vi "I(V) at various fields_MFLI_PK_v4.0_measure X.vi"() -> ()   [LabVIEW 2016]
uses:
  Labview Drivers/MFLI/LabOneLabVIEW-22.02.26577/LabOneLabVIEW-22.02.26577/Zurich Instruments LabOne/Public/Data/ziTypeDemodSampleSingle.ctl
  Labview Drivers/MFLI/LabOneLabVIEW-22.02.26577/LabOneLabVIEW-22.02.26577/Zurich Instruments LabOne/Public/Configure/ziSetValueDouble.vi
  Labview Drivers/MFLI/LabOneLabVIEW-22.02.26577/LabOneLabVIEW-22.02.26577/Zurich Instruments LabOne/Public/Configure/ziGetValueDemodSampleEx.vi
  Labview Drivers/MFLI/LabOneLabVIEW-22.02.26577/LabOneLabVIEW-22.02.26577/Zurich Instruments LabOne/Zurich Instruments LabOne.lvlib
panel:
  out "Time (s)":dbl format="%#_13g"
  in  "Field ramp rate (T/min)":string="0.05"
  in  "Magnetic field stabilization time (s)":dbl=200.0 format="%#_13g"
  in  "Step 2":dbl[](array[numeric])=[0.25] min=-3000.0 max=3000.0 format="%.1e"
  in  "To 2":dbl[](array[numeric])=[6.0] min=-3000.0 max=3000.0 format="%.1e"
  in  "From 2":dbl[](array[numeric])=[8.5] min=-3000.0 max=3000.0 format="%.1e"
  out "Magnetic Field (T)":dbl format="%#_13g"
  in  "Magnet IP Address":string="169.254.46.132"
  out "Demod Sample Out 2":T1={"Timestamps (ticks)"=34359738372, "X (Vrms)"=8.366245757779461e-285, "Y (Vrms)"=1.0096057436928657e-284, "Osc Phase (deg)"=1.69759663376e-313, "Freq (Hz)"=2.607691286315397e-191, "DIO"=4, "AuxIn0 (V)"=0.0, "AuxIn1 (V)"=1.6954746369817e-311, "Trigger"=16}
  out "Demod Sample Out":T1={"Timestamps (ticks)"=34359738372, "X (Vrms)"=8.366245757779461e-285, "Y (Vrms)"=1.0096057436928657e-284, "Osc Phase (deg)"=1.69759663376e-313, "Freq (Hz)"=2.607691286315397e-191, "DIO"=4, "AuxIn0 (V)"=0.0, "AuxIn1 (V)"=1.6954746369817e-311, "Trigger"=16}
  in  "MFLI Current source/Voltage reader":string="DEV4382"
  out "Imeas (A)":dbl=2.528615115e-315
  out "Vmeas (V)":dbl=nan
  in  "Folder":path=path "D:/Pranava/Data/NbO/27-05-2020"
  in  "MFLI stabilization time (s) [> TC]":u32=1
  out "I vs V":cluster{dbl, "Field Reading":dbl}[](graph)=[{nan, "Field Reading"=3.54694038e-315}, {nan, "Field Reading"=2.528615115e-315}]
  out "data":dbl[](array[numeric])=[nan, 2.528615115e-315, 0.0001]
  in  "Step":dbl[](array[numeric])=[0.001, 0.001, 0.001] min=-3000.0 max=3000.0 format="%.1e"
  in  "To":dbl[](array[numeric])=[0.5, -0.5, 0.0] min=-3000.0 max=3000.0 format="%.1e"
  in  "From":dbl[](array[numeric])=[0.0, 0.5, -0.5] min=-3000.0 max=3000.0 format="%.1e"
  in  "file name":string="001_IV_(Nb)STO_7mK_MFLI_MF-MD"
  out "File path":path=path "D:/Pranava/Data/001_IV_(Nb)STO_7mK_MFLI_MF-MD.dat"
  # ".dat"
  # "[Must be less than 0.05]"
  # "Set MFLI Voltage output (V)"
  # "Configure Magnetic field sweep (T)"
types:
  T1 = typedef "Zurich Instruments LabOne.lvlib/ziTypeDemodSampleSingle.ctl" = cluster{"Timestamps (ticks)":u64, "X (Vrms)":dbl, "Y (Vrms)":dbl, "Osc Phase (deg)":dbl, "Freq (Hz)":dbl, "DIO":u32, "AuxIn0 (V)":dbl, "AuxIn1 (V)":dbl, "Trigger":u32}
  T2 = enum16{"open", "replace", "create", "open or create", "replace or create", "replace or create with confirmation"}
  T3 = typedef "Zurich Instruments LabOne.lvlib/ziTypeHandle.ctl" = cluster{"handleValid":bool, "Conn":u64, "Path Prefix":string, "Handle":u64, "Connected":bool, "Clockbase(s)":dbl}
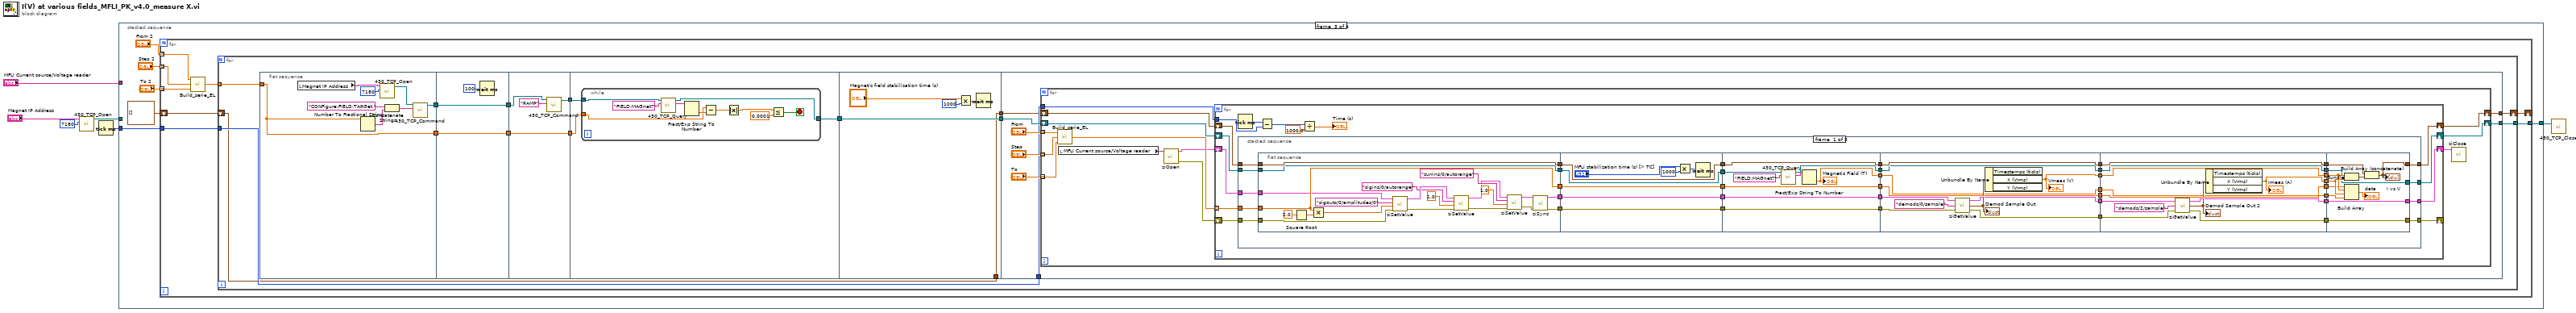
[diagram p0: block diagram]
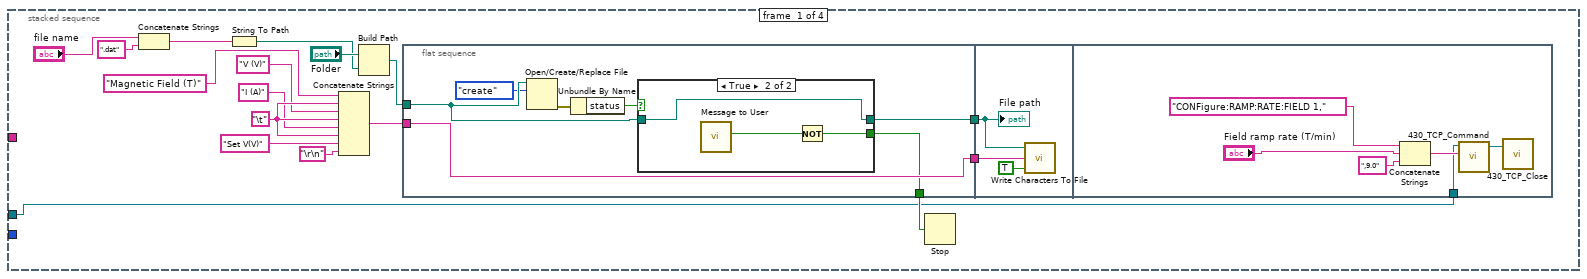
[diagram p2: hidden frame]
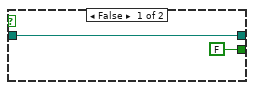
[diagram p3: hidden frame]
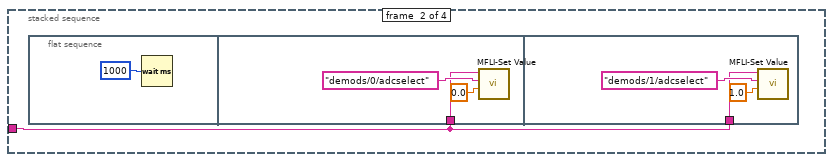
[diagram p4: hidden frame]
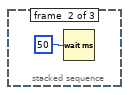
[diagram p5: hidden frame]
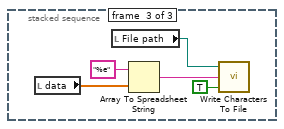
[diagram p6: hidden frame]
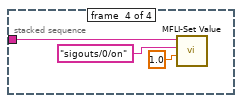
[diagram p7: hidden frame]
diagram:
  n1 = call "430_TCP_Open.vi"("IP Address"="Magnet IP Address", "TCP Port"=7180) -> ("connection ID"=w2:refnum<k5>)  [unwired: 4 in, 2 out]
  n2 = Tick Count (ms)() -> (millisecond timer value=w1:u32)
  n3 = stacked-sequence {
    tunnel: "MFLI Current source/Voltage reader" -> [_ w45 _ w267]
    tunnel: [_ _ w55 _] -> w5
    tunnel: w2 -> [w7 _ _ _]
    tunnel: w1 -> [_ _ w54 _]
    frame #0 {
      w20 = "\t"
      n4 = Concatenate Strings("file name", ".dat" ("string")) -> (w18:string)
      n5 = String To Path(string=w18) -> (path=w9:path)
      n6 = Concatenate Strings("Magnetic Field (T)", w20, "V (V)" ("string"), w20, "I (A)" ("string"), w20, "Set V(V)" ("string"), "\r\n") -> (w19:string)
      n7 = Build Path(base path="Folder", name or relative path=w9) -> (appended path=w8:path)
      n8 = flat-sequence {
        tunnel: w8 -> [w27]
        tunnel: w19 -> [w30]
        tunnel: [w30] -> w23
        tunnel: [w29] -> w16
        tunnel: [w28] -> w22
        tunnel: w23 -> [w37]
        tunnel: w22 -> [w36]
        tunnel: w7 -> [w39]
        frame #0 {
          n9 = Open/Create/Replace File(file path (use dialog)=w27, operation (0:open)=T2."create") -> (error out=w26:errorcluster)  [unwired: 4 in, 2 out]
          n10 = Unbundle By Name(w26) -> ("status"=w24:bool)
          n11 = case shown="True" w24 {
            tunnel: [FALSE ("Yes") w34] -> w29
            tunnel: [w31 w33] -> w28
            tunnel: w27 -> [w31 w33]
            frame False {
            }
            frame True {
              n12 = call "Message to User"() -> ("Yes"=w35:bool)  [unwired: 10 in, 1 out]
              n13 = Not(x=w35) -> (.not. x?=w34:bool)
            }
          }
        }
        frame #1 {
          n14 = call <vilib>:"Write Characters To File.vi"("append to file? (new file:F)"=TRUE, "character string"=w37, "file path (dialog if empty)"=w36) -> ()  [unwired: 2 in, 1 out]
          "File path" <- w36
        }
        frame #2 {
          n15 = Concatenate Strings("CONFigure:RAMP:RATE:FIELD 1," ("String"), "Field ramp rate (T/min)", ",9.0") -> (w40:string)
          n16 = call "430_TCP_Command.vi"("Command"=w40, "connection ID"=w39) -> ("connection ID out"=w44:refnum<k5>)  [unwired: 2 in, 2 out]
          n17 = call "430_TCP_Close.vi"("connection ID"=w44) -> ()  [unwired: 1 in, 2 out]
        }
      }
      n18 = Stop(stop? (T)=w16) -> ()
    }
    frame #1 {
      n19 = flat-sequence {
        tunnel: w45 -> [w47]
        tunnel: w45 -> [w50]
        frame #0 {
          n20 = Wait (ms)(milliseconds to wait=u32 1000) -> ()  [unwired: 1 out]
        }
        frame #1 {
          n21 = call "MFLI-Set Value.vi"("Value"=0.0, "Path"="demods/0/adcselect", "MFLI Current source/Voltage reader"=w47) -> ()  [unwired: 9 in]
        }
        frame #2 {
          n22 = call "MFLI-Set Value.vi"("Value"=1.0, "Path"="demods/1/adcselect", "MFLI Current source/Voltage reader"=w50) -> ()  [unwired: 9 in]
        }
      }
    }
    frame #2 {
      n23 = for {
        tunnel: "From 2" -> [w66] mode=indexing
        tunnel: "To 2" -> [w64] mode=indexing
        tunnel: "Step 2" -> [w65] mode=indexing
        tunnel: [w62] -> w55
        tunnel: w54 -> [w61]
        shift-right: [w59] -> _
        shift-left: cluster{dbl, "Field Reading":dbl}[] [] -> [w60]
        n24 = call "Build_serie_EL.vi"("end value"=w64, "increment"=w65, "start value"=w66) -> ("output array"=w63:dbl[])
        n25 = for {
          tunnel: w63 -> [w80] mode=indexing
          tunnel: [w75] -> w62
          tunnel: w61 -> [w70]
          shift-right: [w67] -> w59
          shift-left: w60 -> [w68]
          n26 = flat-sequence {
            tunnel: w80 -> [w84]
            tunnel: [w85] -> w74
            tunnel: [w84] -> w72
            tunnel: w74 -> [w91]
            tunnel: [w91] -> w73
            tunnel: w72 -> [w90]
            tunnel: [w90] -> w71
            tunnel: w73 -> [w95]
            tunnel: [w93] -> w79
            tunnel: [w92] -> w78
            tunnel: w71 -> [w92]
            tunnel: w79 -> [w98]
            tunnel: w78 -> [w97]
            tunnel: [w96] -> w76
            tunnel: [w110] -> w77
            tunnel: w76 -> [w110]
            tunnel: [w109] -> w69
            tunnel: w68 -> [w109]
            tunnel: w77 -> [w118]
            tunnel: [w117] -> w75
            tunnel: w70 -> [w116]
            tunnel: w69 -> [w115]
            tunnel: [w114] -> w67
            frame #0 {
              n27 = local read "Magnet IP Address"() -> (w82:string)
              n28 = Number To Fractional String(number=w84) -> (F-format string=w86:string)  [unwired: 3 in]
              n29 = call "430_TCP_Open.vi"("IP Address"=w82, "TCP Port"=7180) -> ("connection ID"=w81:refnum<k5>)  [unwired: 4 in, 2 out]
              n30 = Concatenate Strings("CONFigure:FIELD:TARGet " ("String"), w86) -> (w88:string)
              n31 = call "430_TCP_Command.vi"("Command"=w88, "connection ID"=w81) -> ("connection ID out"=w85:refnum<k5>)  [unwired: 2 in, 2 out]
            }
            frame #1 {
              n32 = Wait (ms)(milliseconds to wait=100) -> ()  [unwired: 1 out]
            }
            frame #2 {
              n33 = call "430_TCP_Command.vi"("Command"="RAMP", "connection ID"=w95) -> ("connection ID out"=w93:refnum<k5>)  [unwired: 2 in, 2 out]
            }
            frame #3 {
              n34 = while {
                tunnel: w98 -> [w108]
                tunnel: w97 -> [w103]
                tunnel: [w99] -> w96
                stop <- w101 stop-if-true
                n35 = call "430_TCP_Query.vi"("Command"="FIELD:MAGnet?" ("String"), "connection ID"=w108) -> ("Response"=w107:string, "connection ID out"=w99:refnum<k5>)  [unwired: 5 in, 3 out]
                n36 = Fract/Exp String To Number(string=w107) -> (number=w104:dbl)  [unwired: 3 in, 1 out]
                n37 = Subtract(x=w103, y=w104) -> (x-y=w106:dbl)
                n38 = Absolute Value(x=w106) -> (abs(x)=w105:dbl)
                n39 = Less Or Equal?(x=w105, y=0.0001) -> (x <= y?=w101:bool)
              }
            }
            frame #4 {
              n40 = Multiply(x="Magnetic field stabilization time (s)", y=1000) -> (x*y=w112:dbl)
              n41 = Wait (ms)(milliseconds to wait=w112) -> ()  [unwired: 1 out]
            }
            frame #5 {
              n42 = for {
                tunnel: "From" -> [w131] mode=indexing
                tunnel: "To" -> [w130] mode=indexing
                tunnel: "Step" -> [w129] mode=indexing
                shift-right: [w133] -> w114
                shift-left: w115 -> [w134]
                shift-right: [w125] -> w117
                shift-left: w118 -> [w126]
                tunnel: w116 -> [w124]
                n43 = call "Build_serie_EL.vi"("end value"=w130, "increment"=w129, "start value"=w131) -> ("output array"=w132:dbl[])
                n44 = local read "MFLI Current source/Voltage reader"() -> (w128:string)
                n45 = call "ziOpen.vi"("Address"=w128) -> ("Error Out"=w122:errorcluster, "HandleOut"=w123:T3)  [unwired: 3 in, 1 out]
                n46 = for {
                  tunnel: w132 -> [w148] mode=indexing
                  shift-right: [w146] -> w133
                  shift-left: w134 -> [w147]
                  shift-right: [w143] -> w127
                  shift-left: w123 -> [w145]
                  shift-right: [w142] -> _
                  shift-left: w122 -> [w144]
                  shift-right: [w141] -> w125
                  shift-left: w126 -> [w140]
                  tunnel: w124 -> [w136]
                  n47 = Tick Count (ms)() -> (millisecond timer value=w137:u32)
                  n48 = stacked-sequence {
                    tunnel: w148 -> [w186 _ _]
                    tunnel: w147 -> [w187 _ _]
                    tunnel: [w188 _ _] -> w146
                    tunnel: w145 -> [w181 _ _]
                    tunnel: w144 -> [w180 _ _]
                    tunnel: [w170 _ _] -> w143
                    tunnel: [w169 _ _] -> w142
                    tunnel: [w152 _ _] -> w141
                    tunnel: w140 -> [w151 _ _]
                    frame #0 {
                      n49 = flat-sequence {
                        tunnel: [w209] -> w185
                        tunnel: [w208] -> w184
                        tunnel: w186 -> [w208]
                        tunnel: w187 -> [w209]
                        tunnel: [w190] -> w183
                        tunnel: [w191] -> w182
                        tunnel: w181 -> [w193]
                        tunnel: w180 -> [w192]
                        tunnel: w151 -> [w189]
                        tunnel: [w189] -> w150
                        tunnel: w185 -> [w217]
                        tunnel: [w217] -> w162
                        tunnel: w184 -> [w216]
                        tunnel: [w216] -> w160
                        tunnel: [w215] -> w164
                        tunnel: [w214] -> w166
                        tunnel: w183 -> [w214]
                        tunnel: w182 -> [w215]
                        tunnel: w150 -> [w213]
                        tunnel: [w213] -> w149
                        tunnel: w166 -> [w226]
                        tunnel: [w226] -> w165
                        tunnel: w164 -> [w225]
                        tunnel: [w225] -> w163
                        tunnel: w162 -> [w224]
                        tunnel: [w224] -> w161
                        tunnel: w160 -> [w223]
                        tunnel: [w223] -> w159
                        tunnel: [w220] -> w156
                        tunnel: [w219] -> w155
                        tunnel: w149 -> [w218]
                        tunnel: [w229] -> w179
                        tunnel: [w237] -> w177
                        tunnel: [w236] -> w175
                        tunnel: w165 -> [w233]
                        tunnel: w163 -> [w232]
                        tunnel: w161 -> [w237]
                        tunnel: w159 -> [w236]
                        tunnel: [w231] -> w173
                        tunnel: [w230] -> w172
                        tunnel: [w228] -> w157
                        tunnel: w156 -> [w228]
                        tunnel: w155 -> [w227]
                        tunnel: [w227] -> w153
                        tunnel: w179 -> [w241]
                        tunnel: [w241] -> w178
                        tunnel: w177 -> [w249]
                        tunnel: [w249] -> w176
                        tunnel: w175 -> [w248]
                        tunnel: [w248] -> w174
                        tunnel: w173 -> [w245]
                        tunnel: w172 -> [w244]
                        tunnel: [w243] -> w171
                        tunnel: [w242] -> w168
                        tunnel: [w240] -> w167
                        tunnel: [w239] -> w158
                        tunnel: w157 -> [w239]
                        tunnel: [w238] -> w154
                        tunnel: w153 -> [w238]
                        tunnel: w178 -> [w259]
                        tunnel: [w258] -> w188
                        tunnel: w176 -> [w257]
                        tunnel: w174 -> [w256]
                        tunnel: [w255] -> w170
                        tunnel: w171 -> [w255]
                        tunnel: [w254] -> w169
                        tunnel: w168 -> [w254]
                        tunnel: w167 -> [w253]
                        tunnel: w158 -> [w251]
                        tunnel: w154 -> [w250]
                        tunnel: [w250] -> w152
                        frame #0 {
                          n50 = Square Root(x=2.0) -> (sqrt(x)=w207:dbl)
                          n51 = Multiply(x=w208, y=w207) -> (x*y=w204:dbl)
                          n52 = call-poly "ziSetValue.vi"("Error In"=w192, "Value"=w204, "Path"="sigouts/0/amplitudes/0", "Handle In"=w193) -> ("Error Out"=w200:errorcluster, "Handle Out"=w203:T3)  [unwired: 1 in]
                          n53 = call-poly "ziSetValue.vi"("Error In"=w200, "Value"=1.0, "Path"="sigins/0/autorange", "Handle In"=w203) -> ("Error Out"=w196:errorcluster, "Handle Out"=w197:T3)  [unwired: 1 in]
                          n54 = call-poly "ziSetValue.vi"("Error In"=w196, "Value"=1.0, "Path"="currins/0/autorange", "Handle In"=w197) -> ("Error Out"=w194:errorcluster, "Handle Out"=w195:T3)  [unwired: 1 in]
                          n55 = call "ziSync.vi"("Handle In"=w195, "Error In"=w194) -> ("Handle Out"=w191:T3, "Error Out"=w190:errorcluster)  [unwired: 12 in]
                        }
                        frame #1 {
                          n56 = Multiply(x="MFLI stabilization time (s) [> TC]", y=1000) -> (x*y=w211:u32)
                          n57 = Wait (ms)(milliseconds to wait=w211) -> ()  [unwired: 1 out]
                        }
                        frame #2 {
                          n58 = call "430_TCP_Query.vi"("Command"="FIELD:MAGnet?" ("String"), "connection ID"=w218) -> ("Response"=w222:string, "connection ID out"=w219:refnum<k5>)  [unwired: 5 in, 3 out]
                          n59 = Fract/Exp String To Number(string=w222) -> (number=w220:dbl)  [unwired: 3 in, 1 out]
                          "Magnetic Field (T)" <- w220
                        }
                        frame #3 {
                          n60 = call-poly "ziGetValue.vi"("error in"=w233, "Path"="demods/0/sample", "Handle In"=w232) -> ("error out"=w230:errorcluster, "Demod Sample Out"=w234:T1, "Handle Out"=w231:T3)
                          "Demod Sample Out" <- w234
                          n61 = Unbundle By Name(w234) -> ("X (Vrms)"=w229:dbl)  [unwired: 2 out]
                          "Vmeas (V)" <- w229
                        }
                        frame #4 {
                          n62 = call-poly "ziGetValue.vi"("error in"=w244, "Path"="demods/2/sample", "Handle In"=w245) -> ("error out"=w242:errorcluster, "Demod Sample Out"=w246:T1, "Handle Out"=w243:T3)
                          "Demod Sample Out 2" <- w246
                          n63 = Unbundle By Name(w246) -> ("X (Vrms)"=w240:dbl)  [unwired: 2 out]
                          "Imeas (A)" <- w240
                        }
                        frame #5 {
                          n64 = Bundle("X (Vrms)"=w259, "X (Vrms)"=w253) -> (w252:cluster{"X (Vrms)":dbl, "X (Vrms)":dbl})  [unwired: 1 in]
                          n65 = Build Array(w251, w259, w253, w256) -> (→"data":dbl[])
                          n66 = Build Array (concatenate)(w257, w252) -> (w258:cluster{"X (Vrms)":dbl, "X (Vrms)":dbl}[])
                          "I vs V" <- w258
                        }
                      }
                    }
                    frame #1 {
                      n67 = Wait (ms)(milliseconds to wait=u32 50) -> ()  [unwired: 1 out]
                    }
                    frame #2 {
                      n68 = local read "data"() -> (w262:dbl[])
                      n69 = local read "File path"() -> (w264:path)
                      n70 = Array To Spreadsheet String(array=w262, 3:"%e" ("format string")) -> (spreadsheet string=w265:string)  [unwired: 1 in]
                      n71 = call <vilib>:"Write Characters To File.vi"("append to file? (new file:F)"=TRUE, "character string"=w265, "file path (dialog if empty)"=w264) -> ()  [unwired: 2 in, 1 out]
                    }
                  }
                  n72 = Subtract(x=w137, y=w136) -> (x-y=w139:u32)
                  n73 = Divide(x=w139, y=1000.0) -> (x/y=→"Time (s)":dbl)
                }
                n74 = call "ziClose.vi"("Handle In"=w127) -> ()  [unwired: 1 in, 4 out]
              }
            }
          }
        }
      }
    }
    frame #3 {
      n75 = call "MFLI-Set Value.vi"("Value"=1.0, "Path"="sigouts/0/on", "MFLI Current source/Voltage reader"=w267) -> ()  [unwired: 9 in]
    }
  }
  n76 = call "430_TCP_Close.vi"("connection ID"=w5) -> ()  [unwired: 1 in, 2 out]
